vi "sv_Get Matching Channel Names.vi"(0 "tdms file":refnum<k34>, 5 "group name":string, 7 "channel name substring":string, 9 "channel name substring2":string, 11 "error in (no error)":errorcluster, 12 "separator":string="_") -> (4 "tdms file out":refnum<k34>, 6 "group name out":string, 8 "channel names":string[](array[string]), 15 "error out":errorcluster)   [LabVIEW 2017]
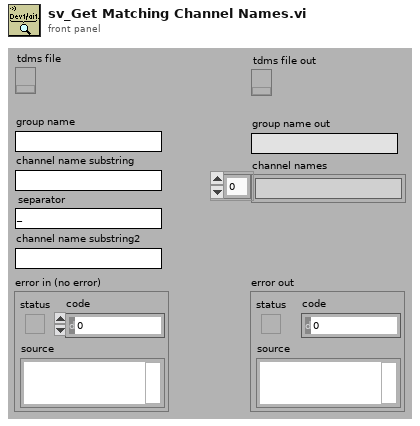
[diagram p1: front panel]
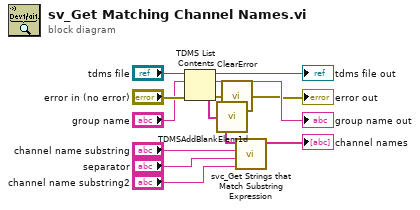
[diagram p0: block diagram]
diagram:
  n1 = TDMS List Contents(4:"error in (no error)", 6:"group name", 7:"tdms file") -> (0:w1:errorcluster, 1:w2:string[], 2:→"group name out":string, 3:→"tdms file out":refnum<k34>)
  n2 = call <vilib>:"TDMSAddBlankElem1d.vi"("input string array"=w2) -> ("output string array with blank element at the beginning"=w7:string[])
  n3 = call <vilib>:"ClearError.vi"("error in (no error)"=w1) -> ("error out"=→"error out":errorcluster)
  n4 = call <vilib>:"svc_Get Strings that Match Substring Expression.vi"("substring 2"="channel name substring2", "separator"="separator", "substring1"="channel name substring", "strings"=w7) -> ("matching strings"=→"channel names":string[])  [unwired: 7 in]
